vi "Test Async Handler Broadcast on Error.vi"(8 "error in (no error)":errorcluster, 11 "Test Case In":refnum<class "Async Handling Test.lvclass">) -> (0 "error out":errorcluster, 3 "Test Case Out":refnum<class "Async Handling Test.lvclass">)   [LabVIEW 2020, in "Async Handling Test.lvclass"]
uses:
  Async Handling Test.lvclass
  C:/Program Files (x86)/National Instruments/LabVIEW 2020/vi.lib/Astemes/LUnit/Test Case.lvclass
  Mock Async Handler Process/Mock Async Handler Process.lvclass
  C:/Git/astemes-triarc-framework/source/Framework/Process/Process.lvclass
  source/Framework/Process/Process.lvclass/Process.ctl
  <vilib>/Astemes/LUnit/Test Case.lvclass/Test Case.ctl
  01074fa8-ee8a-411d-bc8b-fc92c4f90959.vi
  source/Framework/Process/Public/Lifecycle/Get Lifecycle State.vi
  source/Framework/Broadcast Event Helpers/Execution timer.vi
  source/Framework/Process/Private/SubVIs/Wait for finish.vi
  source/Framework/Process/Private/SubVIs/Set Lifecycle State.vi
  source/Framework/Process/Protected/Messaging/Send Message.vi
  <vilib>/Astemes/LUnit/Palette/Pass.vi
  <vilib>/Astemes/LUnit/Palette/Fail.vi
  <vilib>/Astemes/LUnit/Compare Variants.vi
  <vilib>/Astemes/LUnit/Describe Comparison.vi
  <vilib>/Astemes/LUnit/Set Assertion Type.vi
  <vilib>/Utility/error.llb/Clear Errors.vi
  source/Framework/Process/Private/SubVIs/Handle Debug Data.vi
  <vilib>/Astemes/LUnit/Add test result.vi
  <vilib>/Astemes/LUnit/Variant to string.vi
  <vilib>/Utility/High Resolution Relative Seconds.vi
  <vilib>/Astemes/LUnit/LUnit Record Assertion Result.vi
  <vilib>/Astemes/LUnit/LUnit Aggregate Assertion Results.vi
  <vilib>/Astemes/LUnit/Method Result/LUnit Merge Status.vi
  <vilib>/Astemes/LUnit/LUnit Concatenate result strings.vi
  <vilib>/Utility/error.llb/Error Cluster From Error Code.vi
  source/Framework/Broadcast Event Helpers/Dequeue Broadcast Message.vi
  <vilib>/Utility/Data Type/Get Type Information.vi
  <vilib>/Utility/LVClass/Get LV Class Name.vi
  source/Framework/Process/Process.lvclass
  Async Handling Test.lvclass/Async Handling Test.ctl
  source/Framework/Broadcast Event Helpers/Broadcast Event Helpers.lvlib
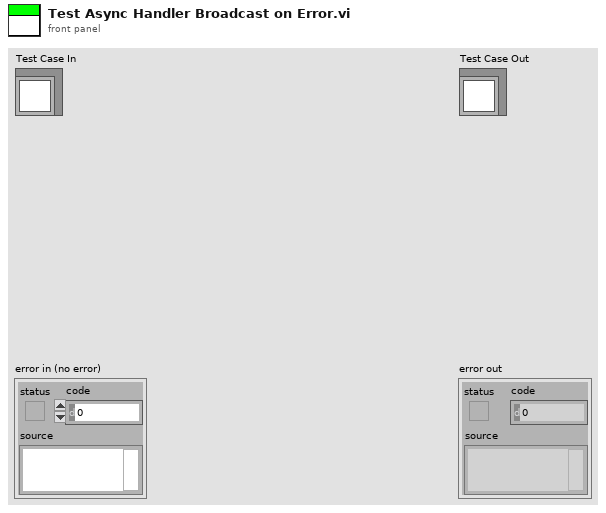
[diagram p1: front panel]
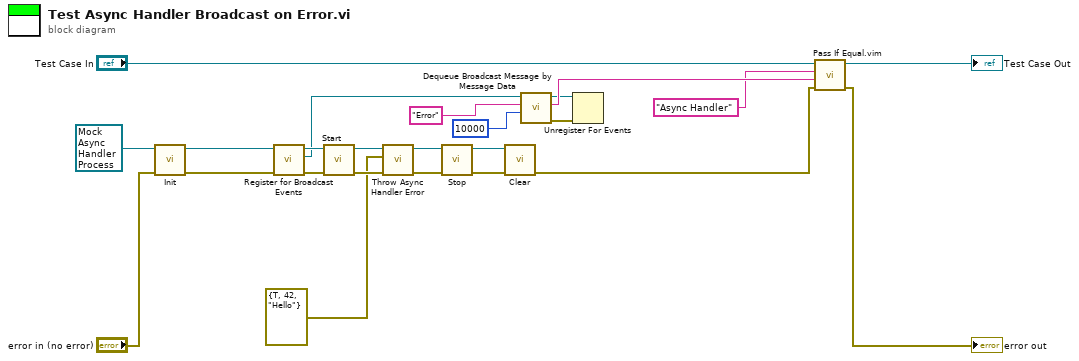
[diagram p0: block diagram]
diagram:
  n1 = call-dynamic "Init.vi"("error in (no error)"="error in (no error)", "Process In"=refnum<class "Mock Async Handler Process.lvclass"> refnum ("Mock Async Handler Process.lvclass")) -> ("error out"=w21:errorcluster, "Process Out"=w17:refnum<class "Mock Async Handler Process.lvclass">)  [unwired: 8 in]
  n2 = call "Register for Broadcast Events.vi"("error in (no error)"=w21, "Process In"=w17) -> ("error out"=w8:errorcluster, "Event Registration Refnum Out"=w6:refnum<event-registration>, "Process Out"=w7:refnum<class "Mock Async Handler Process.lvclass">)  [unwired: 7 in]
  n3 = call "Start.vi"("error in (no error)"=w8, "Process In"=w7) -> ("error out"=w20:errorcluster, "Process Out"=w13:refnum<class "Mock Async Handler Process.lvclass">)  [unwired: 7 in, 1 out]
  n4 = call "Throw Async Handler Error.vi"("error in (no error)"=w20, "Error"=errorcluster {"status"=TRUE, "code"=42, "source"="Hello"}, "Mock Async Handler Process in"=w13) -> ("error out"=w16:errorcluster, "Mock Async Handler Process out"=w15:refnum<class "Mock Async Handler Process.lvclass">)  [unwired: 7 in]
  n5 = call "Stop.vi"("error in (no error)"=w16, "Process In"=w15) -> ("error out"=w18:errorcluster, "Process Out"=w19:refnum<class "Mock Async Handler Process.lvclass">)  [unwired: 7 in, 1 out]
  n6 = call-dynamic "Clear.vi"("error in (no error)"=w18, "Process In"=w19) -> ("error out"=w12:errorcluster)  [unwired: 9 in]
  n7 = call "Dequeue Broadcast Message by Message Data.vi"("Timeout (-1)"=10000, "Message Data"="Error" ("y"), "Event Registration Refnum"=w6) -> ("error out"=w3:errorcluster, "Message"=w11:string, "Event Registration Refnum Out"=w2:refnum<event-registration>)  [unwired: 4 in, 2 out]
  n8 = Unregister For Events(event registration refnum=w2, error in=w3) -> ()  [unwired: 1 out]
  n9 = call "Pass If Equal.vim"("error in (no error)"=w12, "Actual"=w11, "Expected"="Async Handler" ("Message"), "LUnit Test Case In"="Test Case In") -> ("error out"=→"error out":errorcluster, "LUnit Test Case Out"=→"Test Case Out":refnum<class "Async Handling Test.lvclass">)  [unwired: 6 in]
